vi "Receive.vi"(8 "error in (no error)":errorcluster, 10 "Transfer Group in":refnum<class "Transfer Group.lvclass">, 11 "UDP Transceiver in":refnum<class "UDP Transceiver.lvclass">) -> (0 "error out":errorcluster, 2 "Transfer Group out":refnum<class "Transfer Group.lvclass">, 3 "UDP Transceiver out":refnum<class "UDP Transceiver.lvclass">)   [LabVIEW 2017, in "UDP Transceiver.lvlib" / "UDP Transceiver.lvclass"]
uses:
  UDP Transceiver.lvclass
  DSF/Core/Data Sharing Framework Core.lvlibp/Engine/Transfer Group/Transfer Group.lvclass
  UDP Transceiver.lvclass/UDP Transceiver.ctl
  Read Datagram.vi
  Update Transfer.vi
  DSF.Transceiver.UDP.Errors.vi
  UDP Unknown Datagram Error.vi
  UDP Size Mismatch Error.vi
  <vilib>/NI/Memory Manager/VIs/Source.Write.String.vi
  <vilib>/NI/Memory Manager/VIs/Source.Write.Scalar.Base10.vi
  <vilib>/NI/Memory Manager/VIs/Source.Write.Scalar.Base10 (U16).vi
  <vilib>/NI/Memory Manager/VIs/Source.Write.Scalar.Base10 (U64).vi
  DSF/Core/Data Sharing Framework Core.lvlibp/Engine/Transfer Group/Get Transfers.vi
  Create UDP Error.vi
  DSF/Core/Data Sharing Framework Core.lvlibp/Engine/Transfer/Get String Buffer.vi
  DSF/Core/Data Sharing Framework Core.lvlibp/Engine/Internal/Memory/Memory Buffer/Get Memory Buffer Size.vi
  DSF/Core/Data Sharing Framework Core.lvlibp/Engine/Internal/Memory/Memory Buffer/Write Memory Buffer.vi
  DSF/Core/Data Sharing Framework Core.lvlibp/Engine/Internal/Memory/Memory Buffer/Write 1D Array of U8.vi
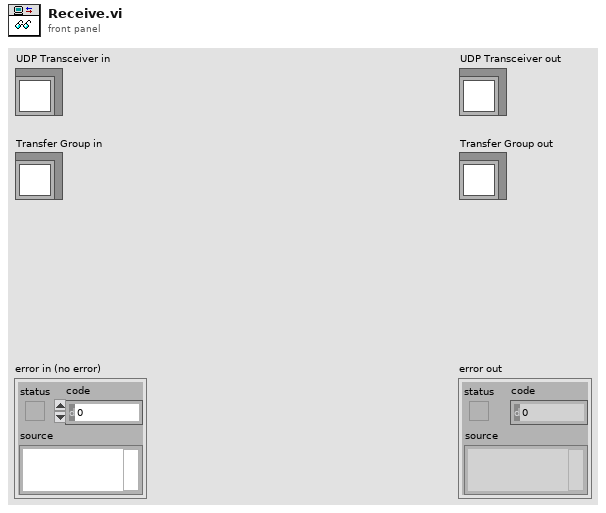
[diagram p1: front panel]
types:
  T1 = typedef "UDP Transceiver.lvlib/UDP Transceiver.lvclass/UDP Transfer Group Parameters.ctl" = cluster{"Rx":T2, "Tx":T4}
  T2 = typedef "UDP Transceiver.lvlib/UDP Transceiver.lvclass/UDP Transfer Group Receive Parameters.ctl" = cluster{"Transfers Rx":T3[], "max size":i32}
  T3 = typedef "UDP Transceiver.lvlib/UDP Transceiver.lvclass/UDP Transfer Receive Parameters.ctl" = cluster{"timeout":i32, "source address":u32, "source port":u16}
  T4 = typedef "UDP Transceiver.lvlib/UDP Transceiver.lvclass/UDP Transfer Group Transmit Parameters.ctl" = cluster{"Transfers Tx":T5[]}
  T5 = typedef "UDP Transceiver.lvlib/UDP Transceiver.lvclass/UDP Transfer Transmit Parameters.ctl" = cluster{"destination port":u16, "destination address":u32}
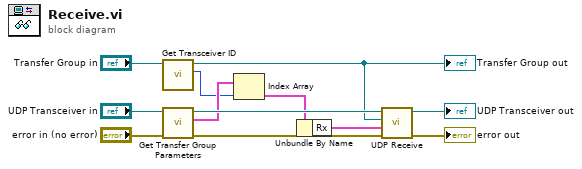
[diagram p0: block diagram]
diagram:
  n1 = call "Get Transceiver ID.vi"("Transfer Group in"="Transfer Group in") -> ("transceiver id"=w8:i32, "Transfer Group out"=w1:refnum<class "Transfer Group.lvclass">)  [unwired: 9 in]
  "Transfer Group out" <- w1
  n2 = call "Get Transfer Group Parameters.vi"("UDP Transceiver in"="UDP Transceiver in") -> ("Transfer Group parameters"=w9:T1[], "UDP Transceiver out"=w10:refnum<class "UDP Transceiver.lvclass">)  [unwired: 9 in]
  n3 = Index Array(array=w9, index=w8) -> (element=w7:T1)
  n4 = Unbundle By Name(w7) -> ("Rx"=w11:T2)
  n5 = call "UDP Receive.vi"("error in (no error)"="error in (no error)", "Transfer Group Rx parameters"=w11, "Transfer Group"=w1, "UDP Transceiver in"=w10) -> ("error out"=→"error out":errorcluster, "UDP Transceiver out"=→"UDP Transceiver out":refnum<class "UDP Transceiver.lvclass">)  [unwired: 6 in]
